vi "CRYRecall Global.vi"() -> ()   [LabVIEW 2013]
panel:
  in  "Recall Path":path
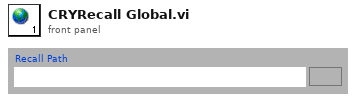
[diagram p1: front panel]
diagram:
